vi "CIET Data Server.vi"() -> ()   [LabVIEW 2017]
uses:
  <vilib>/OPCUA/controls/Data Type.ctl
  <vilib>/OPCUA/controls/Supported Security Policies.ctl
  <vilib>/OPCUA/NI OPC UA Server.lvlib
  <vilib>/OPCUA/NI OPC UA Utility.lvlib
panel:
  out "certificate path 2":path
  out "certificate path":path
  out "error out":errorcluster
  out "CIET node ID":string
  out "server endpoint URL":string
  in  "stop":bool
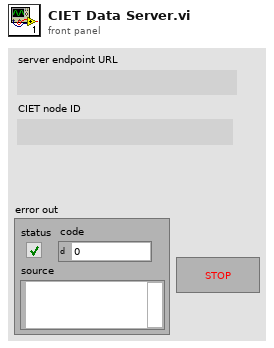
[diagram p1: front panel]
types:
  T1 = typedef "Supported Security Policies.ctl" = cluster{"None":bool, "Sign with Basic128Rsa15":bool, "Sign and Encrypt with Basic128Rsa15":bool, "Sign with Basic256":bool, "Sign and Encrypt with Basic256":bool}
  T2 = typedef "Data Type.ctl" = u16
  T3 = cluster{"name":string, "data type":T2, "access level":u16, "description":string}
  T4 = typedef "OPC UA Server Refnum.ctl" = refnum<k21>
  T5 = typedef "NodeId.ctl" = string
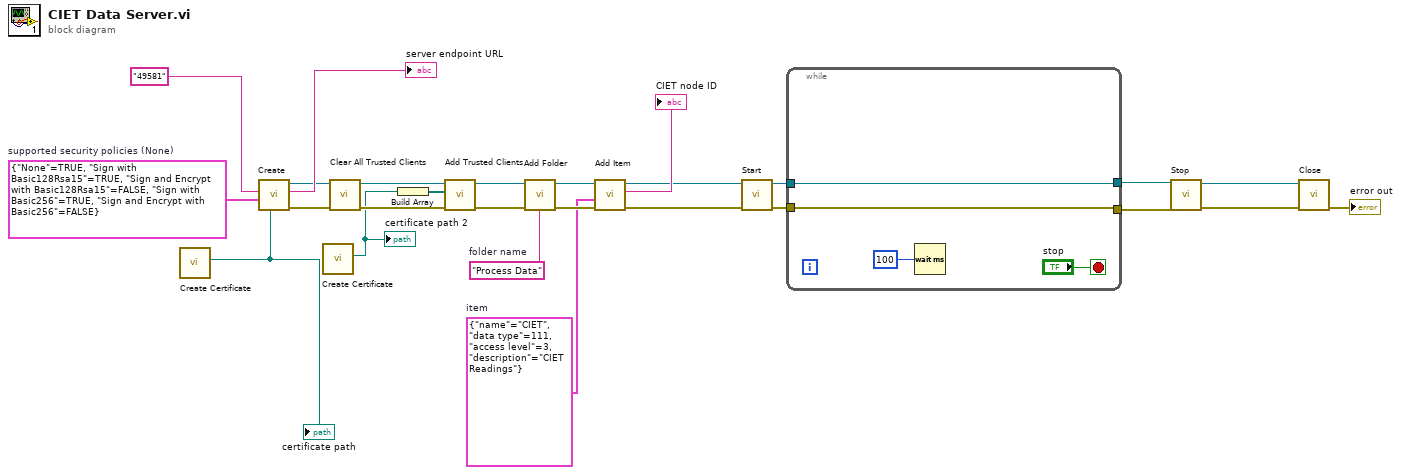
[diagram p0: block diagram]
diagram:
  w13 = T1 {"None"=TRUE, "Sign with Basic128Rsa15"=TRUE, "Sign and Encrypt with Basic128Rsa15"=FALSE, "Sign with Basic256"=TRUE, "Sign and Encrypt with Basic256"=FALSE}  # supported security policies (None)
  w22 = T3 {"name"="CIET", "data type"=111, "access level"=3, "description"="CIET Readings"}  # item
  w23 = "Process Data"  # folder name
  n1 = call <vilib>:"Create Certificate.vi"() -> ("certificate path"=w6:path)  [unwired: 8 in, 3 out]
  "certificate path" <- w6
  n2 = call <vilib>:"Create.vi"("server certificate file"=w6, "supported security policies (None)"=w13, "TCP port (49580)"="49581") -> ("error out"=w9:errorcluster, "server endpoint URL"=→"server endpoint URL":string, "OPC UA server refnum out"=w10:T4)  [unwired: 6 in]
  n3 = call <vilib>:"Create Certificate.vi"() -> ("certificate path"=w5:path)  [unwired: 8 in, 3 out]
  "certificate path 2" <- w5
  n4 = call <vilib>:"Clear All Trusted Clients.vi"("error in (no error)"=w9, "OPC UA server refnum in"=w10) -> ("error out"=w11:errorcluster, "OPC UA server refnum out"=w12:T4)  [unwired: 8 in]
  n5 = Build Array(w5) -> (w4:path[])
  n6 = call <vilib>:"Add Trusted Clients.vi"("error in (no error)"=w11, "trusted client certificates"=w4, "OPC UA server refnum in"=w12) -> ("error out"=w7:errorcluster, "OPC UA server refnum out"=w8:T4)  [unwired: 7 in]
  n7 = call <vilib>:"Add Folder.vi"("error in (no error)"=w7, "folder name"=w23, "OPC UA server refnum in"=w8) -> ("error out"=w25:errorcluster, "OPC UA server refnum out"=w26:T4)  [unwired: 5 in, 1 out]
  n8 = call <vilib>:"Add Item.vi"("error in (no error)"=w25, "item"=w22, "OPC UA server refnum in"=w26) -> ("error out"=w2:errorcluster, "item node ID"=→"CIET node ID":T5, "OPC UA server refnum out"=w3:T4)  [unwired: 4 in, 1 out]
  n9 = call <vilib>:"Start.vi"("error in (no error)"=w2, "OPC UA server refnum in"=w3) -> ("error out"=w19:errorcluster, "OPC UA server refnum out"=w20:T4)  [unwired: 7 in, 1 out]
  n10 = while {
    tunnel: [w30] -> w17
    tunnel: w20 -> [w30]
    tunnel: [w29] -> w18
    tunnel: w19 -> [w29]
    stop <- "stop" stop-if-true
    n11 = Wait (ms)(milliseconds to wait=u32 100) -> ()  [unwired: 1 out]
  }
  n12 = call <vilib>:"Stop.vi"("error in (no error)"=w18, "OPC UA server refnum in"=w17) -> ("error out"=w15:errorcluster, "OPC UA server refnum out"=w16:T4)  [unwired: 8 in]
  n13 = call <vilib>:"Close.vi"("error in (no error)"=w15, "OPC UA server refnum in"=w16) -> ("error out"=→"error out":errorcluster)  [unwired: 9 in]
